vi "sub_main_PXI-5110.vi"(8 "error in":errorcluster) -> (0 "error out":errorcluster)   [LabVIEW 2021]
uses:
  ctrl/create-rw-close.ctl
  ctrl/hw-lists.ctl
  ctrl/ini-stop-read.ctl
  ctrl/5110_q.ctl
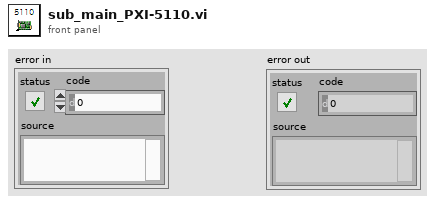
[diagram p1: front panel]
types:
  T1 = typedef "hw-lists.ctl" = enum16{"PXIe-5110", "PXIe-5413", "PXIe-2530", "DS1202"}
  T2 = typedef "create-rw-close.ctl" = enum16{"create", "read", "write", "close"}
  T3 = enum16{"init", "config", "trigger", "read", "close"}
  T4 = typedef "5110_q.ctl" = enum16{"create", "read", "write", "close"}
  T5 = typedef "ini-stop-read.ctl" = enum16{"init", "stop", "read"}
  T6 = typedef "run-check-stop.ctl" = enum16{"run", "check", "stop"}
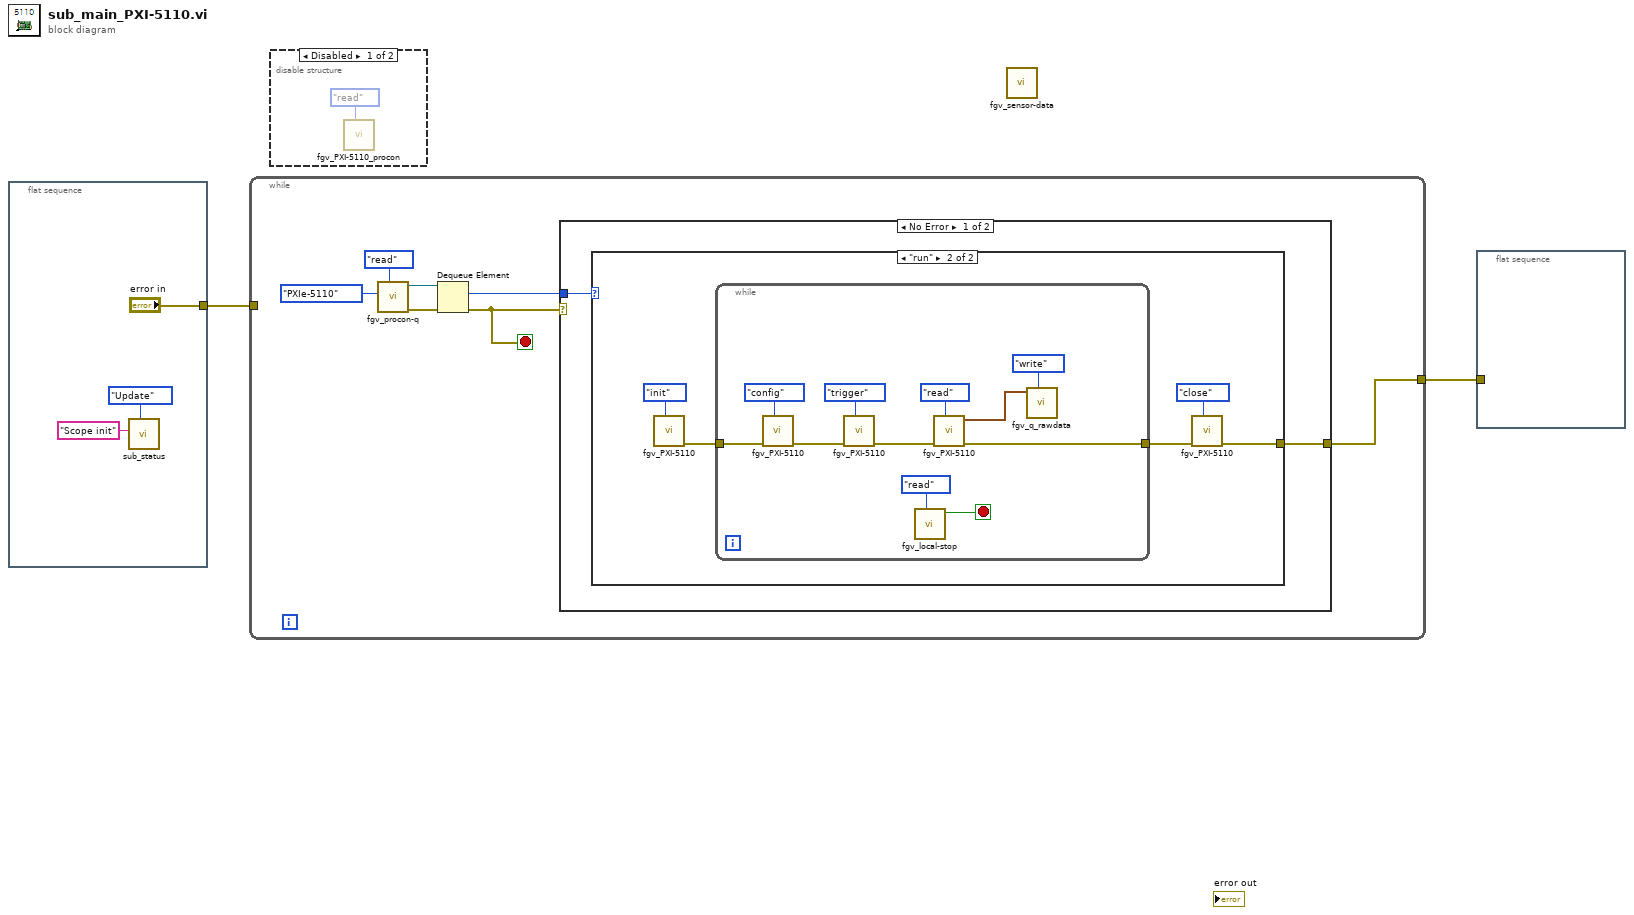
[diagram p0: block diagram]
diagram:
  n1 = flat-sequence {
    tunnel: ["error in"] -> w1
    frame #0 {
      n2 = call "sub_status.vi"("Mode"=enum16{"Initial", "Update", "Clear"}."Update", "title"="Scope init") -> ()  [unwired: 9 in, 1 out]
    }
  }
  n3 = while {
    tunnel: w1 -> [_]
    tunnel: [w10] -> w2
    stop <- w12 stop-if-true
    n4 = call "fgv_procon-q.vi"("cmd 2"=create-rw-close."read", "hw lists"=hw-lists."PXIe-5110") -> ("error out"=w6:errorcluster, "ref"=w7:refnum<queue>)  [unwired: 7 in, 1 out]
    n5 = Dequeue Element(queue=w7, error in (no error)=w6) -> (element=w11:T6, error out=w12:errorcluster)  [unwired: 1 in, 2 out]
    n6 = case shown="No Error" w12 {
      tunnel: w11 -> [w14 _]
      tunnel: [w13 _] -> w10
      frame No Error {
        n7 = case shown="\"run\"" w14 {
          tunnel: [_ w15] -> w13
          frame "check", Default {
          }
          frame "run" {
            n8 = call "fgv_PXI-5110.vi"("cmd"=T3."init") -> ("error out"=w17:errorcluster)  [unwired: 9 in, 1 out]
            n9 = while {
              tunnel: w17 -> [w27]
              tunnel: [w24] -> w16
              stop <- w22 stop-if-true
              n10 = call "fgv_PXI-5110.vi"("cmd"=T3."config", "error in"=w27) -> ("error out"=w26:errorcluster)  [unwired: 8 in, 1 out]
              n11 = call "fgv_PXI-5110.vi"("cmd"=T3."trigger", "error in"=w26) -> ("error out"=w25:errorcluster)  [unwired: 8 in, 1 out]
              n12 = call "fgv_local-stop.vi"("cmd"=ini-stop-read."read") -> ("stop"=w22:bool)  [unwired: 10 in]
              n13 = call "fgv_PXI-5110.vi"("cmd"=T3."read", "error in"=w25) -> ("error out"=w24:errorcluster, "wfm"=w20:waveform(dbl))  [unwired: 8 in]
              n14 = call "fgv_q_rawdata.vi"("cmd"=5110_q."write", "wfm"=w20) -> ()  [unwired: 8 in, 2 out]
            }
            n15 = call "fgv_PXI-5110.vi"("cmd"=T3."close", "error in"=w16) -> ("error out"=w15:errorcluster)  [unwired: 8 in, 1 out]
          }
        }
      }
      frame Error {
      }
    }
  }
  n16 = disable-structure shown="Disabled" {
    frame Disabled {
      n17 = call "fgv_PXI-5110_procon.vi"("cmd"=create-rw-close."read") -> ()  [unwired: 9 in, 2 out]
    }
    frame Enabled {
    }
  }
  n18 = call "fgv_sensor-data.vi"() -> ()  [unwired: 12 in]
  n19 = flat-sequence {
    tunnel: w2 -> [_]
    frame #0 {
    }
  }
